vi "SplitArrStrIndex.vi"(5 "ArrayStr":string) -> (0 "ArrayIndex":u64[](array[numeric]), 1 "ArrayName":string)   [LabVIEW 2016]
uses:
  <vilib>/regexp/Match Regular Expression.xnode
panel:
  # "Array string: e.g. Array[2][3][4][...]"
  # "Split index as a array"
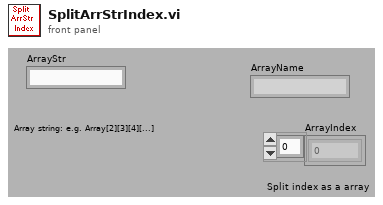
[diagram p1: front panel]
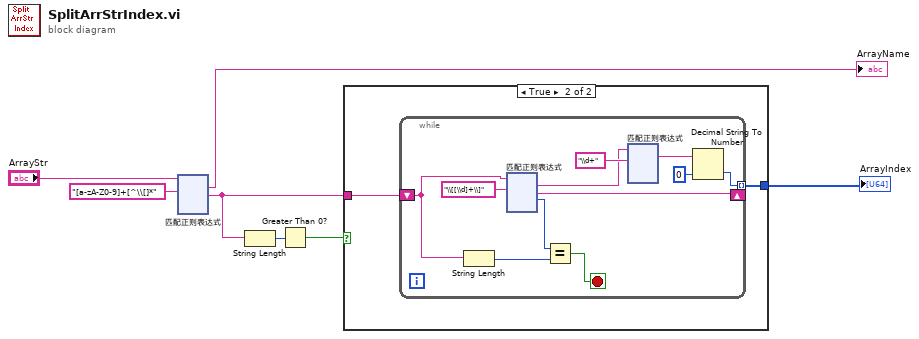
[diagram p0: block diagram]
diagram:
  n1 = xnode "匹配正则表达式"("input string"="ArrayStr", "regular expression"="[a-zA-Z0-9]+[^\\[]*" ("正则表达式")) -> ("whole match"=→"ArrayName":string, "after match"=w4:string)  [unwired: 2 in, 5 out]
  n2 = String Length(string=w4) -> (length=w3:i32)
  n3 = Greater Than 0?(x=w3) -> (x > 0?=w2:bool)
  n4 = case shown="True" w2 {
    tunnel: [_ w9] -> w1
    tunnel: w4 -> [_ w8]
    frame False {
    }
    frame True {
      n5 = while {
        tunnel: [w11] -> w9 mode=indexing
        shift-right: [w16] -> _
        shift-left: w8 -> [w15]
        stop <- w17 stop-if-true
        n6 = String Length(string=w15) -> (length=w18:i32)
        n7 = xnode "匹配正则表达式"("input string"=w15, "regular expression"="\\[[\\d]+\\]" ("正则表达式")) -> ("whole match"=w13:string, "after match"=w16:string, "offset past match"=w19:i32)  [unwired: 2 in, 4 out]
        n8 = Equal?(x=w19, y=w18) -> (x = y?=w17:bool)
        n9 = xnode "匹配正则表达式"("input string"=w13, "regular expression"="\\d+" ("正则表达式")) -> ("whole match"=w12:string)  [unwired: 2 in, 6 out]
        n10 = Decimal String To Number(string=w12, default (0L)=u64 0 ("默认(0 I32)")) -> (number=w11:u64)  [unwired: 2 out]
      }
    }
  }
  "ArrayIndex" <- w1
